vi "KG set run.vi"(8 "Fehler (Eingang, kein Fehler)":errorcluster, 10 "run":bool, 11 "VISA-Ressourcenname":refnum<visa-resource-name>) -> (0 "Fehler (Ausgang)":errorcluster, 2 "Kommando gesendet":string, 3 "VISA-Ressourcenname (Ausgang)":refnum<visa-resource-name>)   [LabVIEW 2020, in "Linearisierung v2.lvlib" / "Gasteiler.lvlib" / "HovaCAL_Interface.lvlib" / "KGN.lvlib" / "set.lvlib"]
uses:
  set.lvlib
  KGN.lvlib
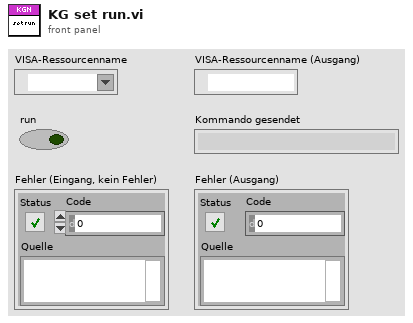
[diagram p1: front panel]
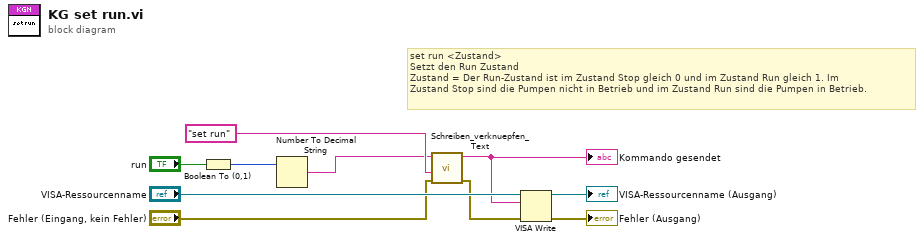
[diagram p0: block diagram]
diagram:
  # "set run <Zustand>\nSetzt den Run Zustand\nZustand = Der Run-Zustand ist im Zustand Stop gleich 0 und im Zustand Run gleich 1. Im\nZustand Stop sind die Pumpen nicht in Betrieb und im Zustand Run sind die Pumpen in Betrieb."
  n1 = Boolean To (0,1)(Boolean="run") -> (0, 1=w6:i16)
  n2 = Number To Decimal String(number=w6) -> (decimal integer string=w1:string)  [unwired: 1 in]
  n3 = call "Schreiben_verknuepfen_Text.vi"("error in (no error)"="Fehler (Eingang, kein Fehler)", "Order"="set run" ("Schreibpuffer"), "parameter"=w1) -> ("error out"=w4:errorcluster, "Verknüpfter String"=w3:string)  [unwired: 7 in]
  "Kommando gesendet" <- w3
  n4 = VISA Write(VISA resource name="VISA-Ressourcenname", write buffer=w3, error in (no error)=w4) -> (VISA resource name out=→"VISA-Ressourcenname (Ausgang)":refnum<visa-resource-name>, error out=→"Fehler (Ausgang)":errorcluster)  [unwired: 1 out]
